vi "Push_Data_to_Server.vi"(2 "Archive File?":bool, 3 "File String":string, 4 "Path of File relative to EnFlo Data Root":path) -> (0 "error out":errorcluster)   [LabVIEW 2011]
uses:
  Anemometry/Anemometry Sub Vis/Globals/Constants_global.vi
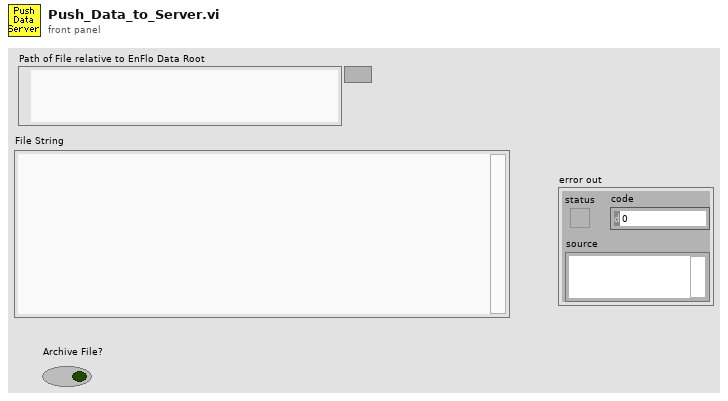
[diagram p1: front panel]
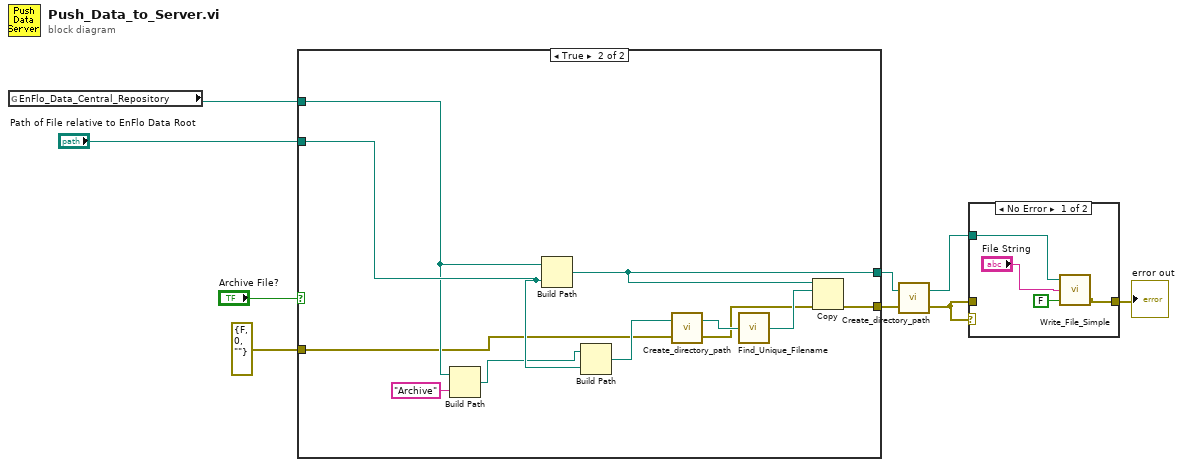
[diagram p0: block diagram]
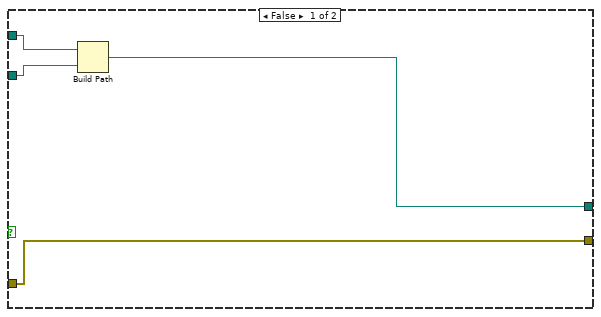
[diagram p2: hidden frame]
diagram:
  n1 = global read "Constants_global.vi" "EnFlo_Data_Central_Repository"() -> (w7:path)
  n2 = case shown="True" "Archive File?" {
    tunnel: w7 -> [w13 w18]
    tunnel: "Path of File relative to EnFlo Data Root" -> [w12 w20]
    tunnel: [w10 w16] -> w4
    tunnel: errorcluster {"status"=FALSE, "code"=0, "source"=""} ("error out") -> [w10 w15]
    tunnel: [w11 w14] -> w2
    frame False {
      n3 = Build Path(base path=w13, name or relative path=w12) -> (appended path=w11:path)
    }
    frame True {
      n4 = Build Path(base path=w18, name or relative path="Archive") -> (appended path=w17:path)
      n5 = Build Path(base path=w18, name or relative path=w20) -> (appended path=w14:path)
      n6 = Build Path(base path=w17, name or relative path=w20) -> (appended path=w23:path)
      n7 = call "Create_directory_path.vi"("error in (no error)"=w15, "Path name"=w23) -> ("error out"=w21:errorcluster, "Path name Out"=w22:path)
      n8 = call "Find_Unique_Filename.vi"("Path In"=w22) -> ("Unique Path Out"=w24:path)  [unwired: 2 in]
      n9 = Copy(8:w21, 10:w24, 11:w14) -> (0:w16:errorcluster)  [unwired: 2 in, 2 out]
    }
  }
  n10 = call "Create_directory_path.vi"("error in (no error)"=w4, "Path name"=w2) -> ("error out"=w3:errorcluster, "Path name Out"=w1:path)
  n11 = case shown="No Error" w3 {
    tunnel: [w27 w29] -> w9
    tunnel: w1 -> [w26 _]
    tunnel: w3 -> [_ w29]
    frame No Error {
      n12 = call "Write_File_Simple.vi"("append to file? (new file:F)"=FALSE, "character string"="File String", "file path"=w26) -> ("error out"=w27:errorcluster)  [unwired: 1 out]
    }
    frame Error {
    }
  }
  "error out" <- w9
